vi "Wait.vi"(7 "Wait (ms)":u32, 10 "ErrorIn":errorcluster) -> (2 "ErrorOut":errorcluster)   [LabVIEW 2018]
doc: "This waits the specified number of milliseconds (defined by <B>Wait (ms))</B>.\n\nIt is useful to enforce dataflow because it includes <B>ErrorIn</B> and <B>ErrorOut</B>, although these are not affected by this VI.\n\nCopyright © 2019 Epimedia, Inc. All Rights Reserved.\n\nThe Epimedia Application Library is Copyright © 2009-2017 Epimedia, Inc. \nAll Rights Reserved. Used under license."
panel:
  # "Copyright © 2019 Epimedia, Inc. All Rights Reserved.\n\nThe Epimedia Application Library is Copyright © 2009-2017 Epimedia, Inc. \nAll Rights Reserved. Used under license."
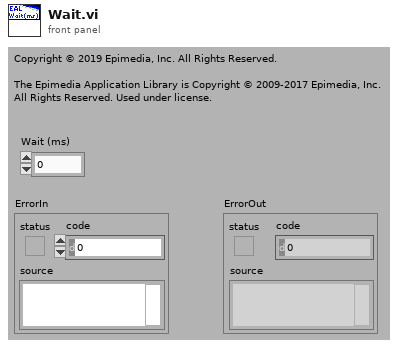
[diagram p1: front panel]
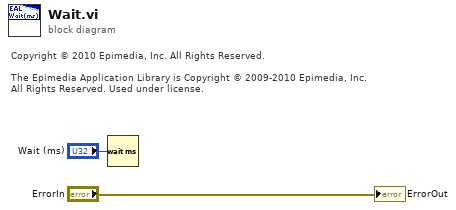
[diagram p0: block diagram]
diagram:
  # "Copyright © 2010 Epimedia, Inc. All Rights Reserved.\n\nThe Epimedia Application Library is Copyright © 2009-2010 Epimedia, Inc. \nAll Rights Reserved. Used under license."
  n1 = Wait (ms)(milliseconds to wait="Wait (ms)") -> ()  [unwired: 1 out]
  "ErrorOut" <- "ErrorIn"
